vi "test_ping.vi"() -> ()   [LabVIEW 2013]
panel:
  out "chaîne en sortie":string
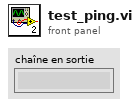
[diagram p1: front panel]
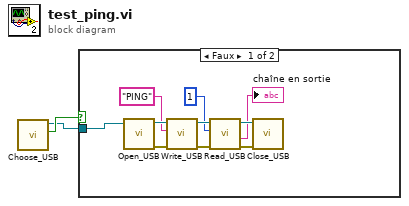
[diagram p0: block diagram]
diagram:
  n1 = call "Choose_USB.vi"() -> ("Annulé?"=w2:bool, "Nom de ressource VISA en sortie"=w1:refnum<visa-resource-name>)  [unwired: 10 in]
  n2 = case shown="Faux" w2 {
    tunnel: w1 -> [w3 _]
    frame False {
      n3 = call "Open_USB.vi"("Nom de ressource VISA"=w3) -> ("error out"=w11:errorcluster, "Nom de ressource VISA ouverte"=w12:refnum<visa-resource-name>)  [unwired: 9 in]
      n4 = call "Write_USB.vi"("entrée d'erreur (pas d'erreur)"=w11, "buffer d'écriture"="PING", "Nom de ressource VISA"=w12) -> ("sortie d'erreur"=w7:errorcluster, "Nom de ressource VISA en sortie"=w9:refnum<visa-resource-name>)  [unwired: 7 in]
      n5 = call "Read_USB.vi"("entrée d'erreur (pas d'erreur)"=w7, "timeout (0)"=u32 1, "Nom de ressource VISA"=w9) -> ("sortie d'erreur"=w5:errorcluster, "chaîne en sortie"=→"chaîne en sortie":string, "Nom de ressource VISA en sortie"=w6:refnum<visa-resource-name>)  [unwired: 6 in]
      n6 = call "Close_USB.vi"("entrée d'erreur (pas d'erreur)"=w5, "Nom de ressource VISA"=w6) -> ()  [unwired: 9 in, 1 out]
    }
    frame True {
    }
  }
